vi "Pressure Sensor-Direct.vi"() -> ()   [LabVIEW 2009]
uses:
  <vilib>/NXT/Block Support/NXT_InputPort.ctl
  <vilib>/NXT/Subs/LVHSConnector.ctl
panel:
  out "NXT dup":T1={"error"={"status"=FALSE, "code"=0, "source"=""}, "address"="", "NXT #"=-1, "Show Error"=TRUE}
  in  "NXT":T1={"error"={"status"=FALSE, "code"=0, "source"=""}, "address"="", "NXT #"=-1, "Show Error"=TRUE}
  in  "stop":bool
  out "Pressure Guage (psi)":u8(slide)=5 scale=0.0..100.0
  in  "Input":T2 items=["Port 1", "Port 2", "Port 3", "Port 4"]
  out "Pressure (psi)":i16=40
  # "mindsensors.com\nCopyright (c) 2009 by mindsensors.com\nEmail: info (<at>) mindsensors (<dot>) com\n\nThis program is free software. You can redistribute it and/or modify\nit under the terms of the GNU General Public License as published by\nthe Free Software Foundation; version 3 of the License.\nRead the license at: http://www.gnu.org/licenses/gpl.txt"
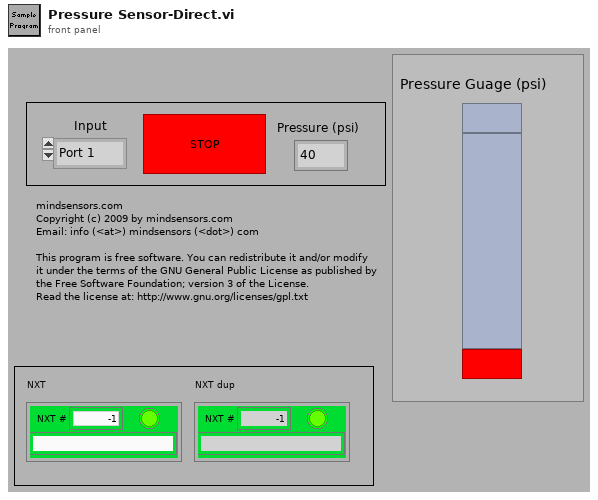
[diagram p1: front panel]
types:
  T1 = typedef "LVHSConnector.ctl" = cluster{"error":errorcluster, "address":string, "NXT #":i32, "Show Error":bool}
  T2 = typedef "NXT_InputPort.ctl" = u8
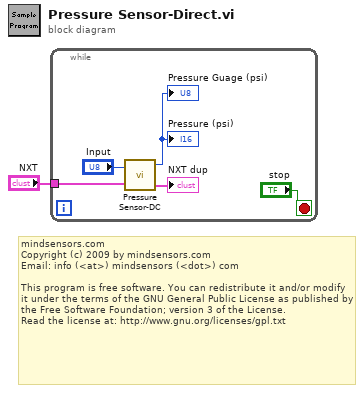
[diagram p0: block diagram]
diagram:
  # "mindsensors.com\nCopyright (c) 2009 by mindsensors.com\nEmail: info (<at>) mindsensors (<dot>) com\n\nThis program is free software. You can redistribute it and/or modify\nit under the terms of the GNU General Public License as published by\nthe Free Software Foundation; version 3 of the License.\nRead the license at: http://www.gnu.org/licenses/gpl.txt"
  n1 = while {
    tunnel: "NXT" -> [w3]
    stop <- "stop" stop-if-true
    n2 = call "Pressure Sensor-DC.vi"("Input Port"="Input", "NXT"=w3) -> ("Scaled Value"=→"Pressure (psi)" →"Pressure Guage (psi)":i16, "NXT dup"=→"NXT dup":T1)  [unwired: 1 out]
  }
